vi "Read Sample Container.vi"(8 "error in (no error)":errorcluster, 11 "Capillary Line in":refnum<class "Capillary Line.lvclass">) -> (0 "error out":errorcluster, 1 "Sample":refnum<class "Sample.lvclass">, 2 "Container":T1, 3 "Capillary Line out":refnum<class "Capillary Line.lvclass">)   [LabVIEW 2015, in "cRIO-Carbondioxide.lvlib" / "CO2-Actor.lvlib" / "Capillary Line.lvclass"]
uses:
  Capillary Line.lvclass
  subs/Sample/Sample.lvclass
  Controls/Sample Container.ctl
  Capillary Line.lvclass/Capillary Line.ctl
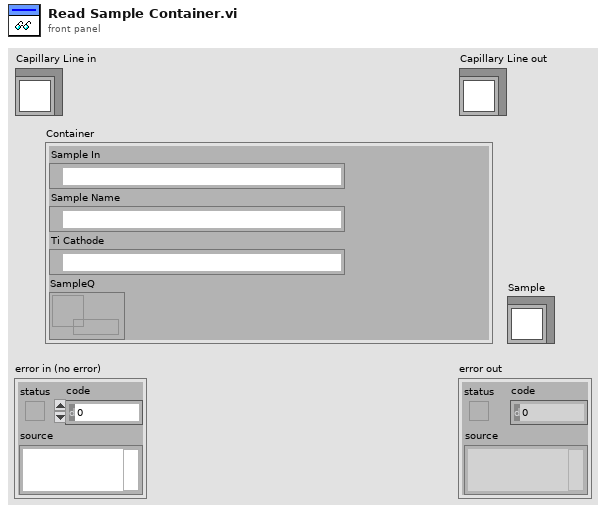
[diagram p1: front panel]
types:
  T1 = typedef "Sample Container.ctl" = cluster{"Sample In":refnum<k21>, "Sample Name":refnum<k21>, "Ti Cathode":refnum<k21>, "SampleQ":refnum<queue>}
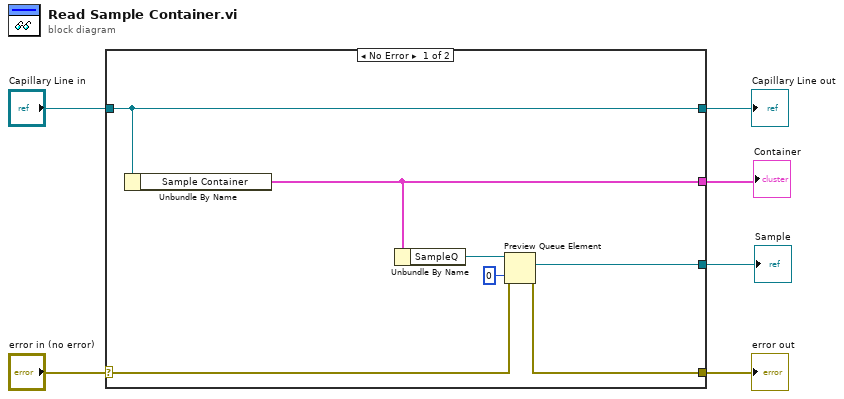
[diagram p0: block diagram]
diagram:
  n1 = case shown="No Error" "error in (no error)" {
    selector: "error in (no error)" -> [w10 w15]
    tunnel: [w9 w15] -> w4
    tunnel: [w13 w14] -> w3
    tunnel: "Capillary Line in" -> [w13 w14]
    tunnel: [w12 _] -> w2
    tunnel: [w7 _] -> w1
    frame No Error {
      n2 = Unbundle By Name(w13) -> ("Sample Container"=w12:T1)
      n3 = Unbundle By Name(w12) -> ("SampleQ"=w11:refnum<queue>)
      n4 = Preview Queue Element(queue=w11, timeout in ms (-1)=0, error in (no error)=w10) -> (element=w7:refnum<class "Sample.lvclass">, error out=w9:errorcluster)  [unwired: 2 out]
    }
    frame Error {
    }
  }
  "error out" <- w4
  "Capillary Line out" <- w3
  "Container" <- w2
  "Sample" <- w1
